vi "Read Matlab Params.vi"(8 "error in (no error)":errorcluster, 10 "Enum":T1(ring), 11 "TrialBasedExperiment in":refnum<class "EyeCalibration.lvclass">) -> (0 "error out":errorcluster, 2 "Matlab Param Array":cluster{"Name":string, "Data":variant}[](array[cluster]), 3 "TrialBasedExperiment out":refnum<class "EyeCalibration.lvclass">)   [LabVIEW 2011, in "EyeCalibration.lvclass"]
uses:
  EyeCalibration.lvclass
  Trial Based Experiment Statechart/MatlabExperiment/MatlabExperiment.lvclass
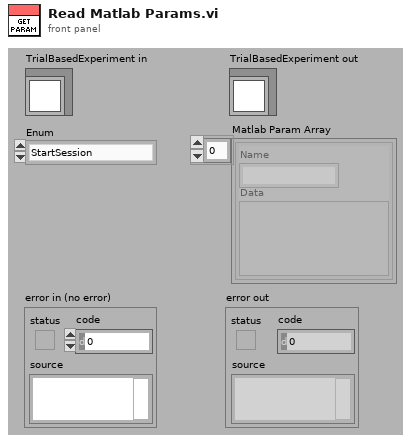
[diagram p1: front panel]
types:
  T1 = enum16{"StartSession", "StartTrial", "ShowStimulus"}
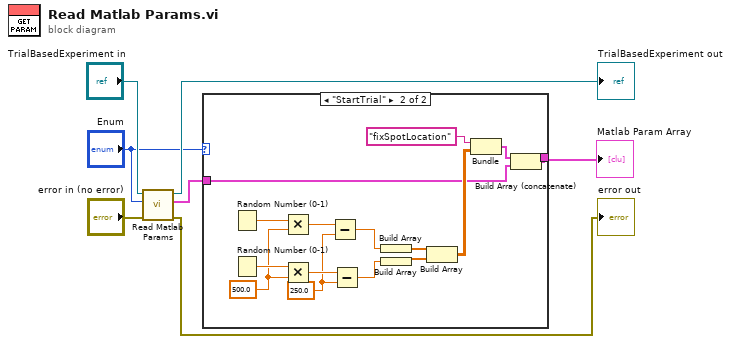
[diagram p0: block diagram]
diagram:
  n1 = call-parent "Read Matlab Params.vi"("error in (no error)"="error in (no error)", "Enum"="Enum", "TrialBasedExperiment in"="TrialBasedExperiment in") -> ("error out"=→"error out":errorcluster, "Matlab Param Array"=w2:cluster{"Name":string, "Data":variant}[], "TrialBasedExperiment out"=→"TrialBasedExperiment out":refnum<class "EyeCalibration.lvclass">)  [unwired: 6 in]
  n2 = case shown="\"StartTrial\"" "Enum" {
    tunnel: w2 -> [w8 w20]
    tunnel: [w8 w19] -> w1
    frame "StartSession", Default {
    }
    frame "StartTrial" {
      w13 = 250.0 ("y")
      w16 = 500.0 ("y")
      n3 = Random Number (0-1)() -> (number: 0 to 1=w18:dbl)
      n4 = Random Number (0-1)() -> (number: 0 to 1=w17:dbl)
      n5 = Multiply(x=w18, y=w16) -> (x*y=w15:dbl)
      n6 = Multiply(x=w17, y=w16) -> (x*y=w14:dbl)
      n7 = Subtract(x=w15, y=w13) -> (x-y=w12:dbl)
      n8 = Subtract(x=w14, y=w13) -> (x-y=w11:dbl)
      n9 = Build Array(w12) -> (w10:dbl[])
      n10 = Build Array(w11) -> (w9:dbl[])
      n11 = Build Array(w10, w9) -> (w23:dbl[][])
      n12 = Bundle("fixSpotLocation", w23) -> (w21:cluster{string, dbl[][]})  [unwired: 1 in]
      n13 = Build Array (concatenate)(w21, w20) -> (w19:cluster{"Name":string, "Data":variant}[])
    }
  }
  "Matlab Param Array" <- w1
